vi "Window-Playback speed entry.vi"() -> (0 "error out":errorcluster, 2 "Frame rate set (fps)":dbl)   [LabVIEW 2013]
doc: "Use this template to create a dialog box with event handling."
uses:
  <vilib>/Utility/miscctls.llb/LVPointTypeDef.ctl
  Globals/gl_Time series viewer globals.vi
  Global Variables/General Globals.vi
panel:
  in  "Use custom FPS":bool
  out "Ind":dbl format="%#.1f FPS"
  in  "Playback speed (FPS)":dbl(slide)=10.0 caption="Playback speed" min=1.0 max=300.0 step=1.0 scale=1.0..300.0
  in  "Cancel":bool
  in  "OK":bool
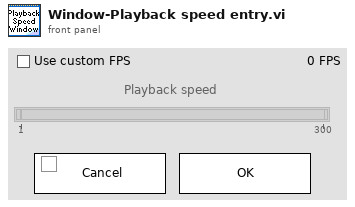
[diagram p1: front panel]
types:
  T1 = typedef "LVPointTypeDef.ctl" = cluster{"Horizontal":i16, "Vertical":i16}
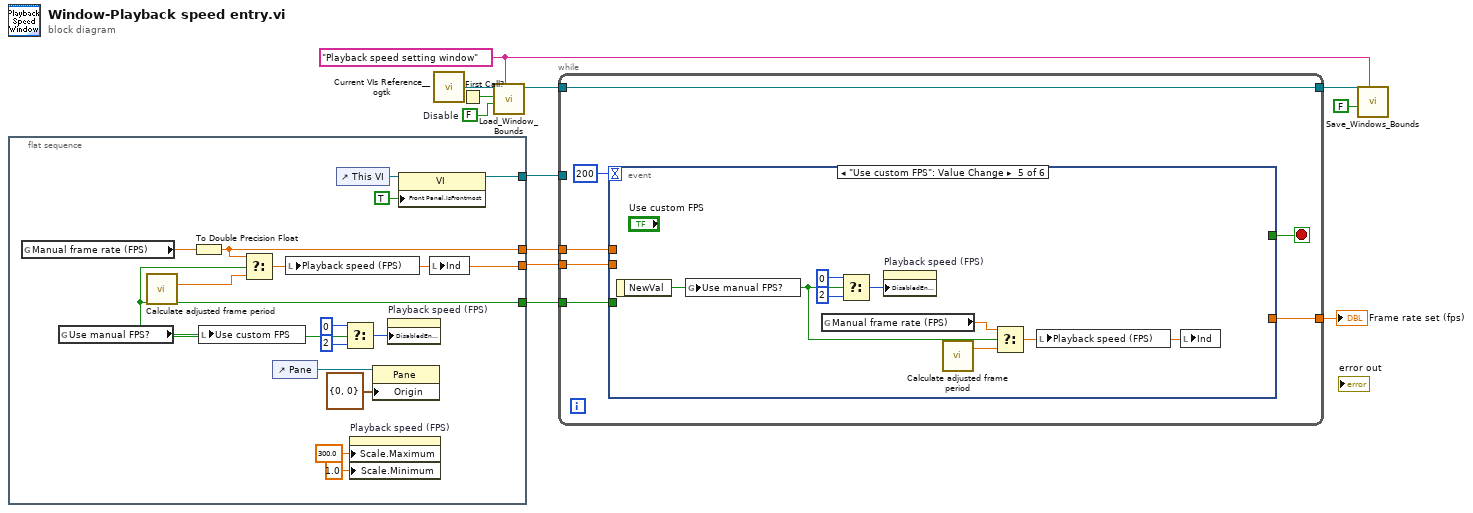
[diagram p0: block diagram]
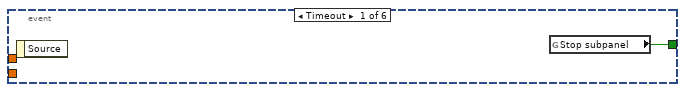
[diagram p2: hidden frame]
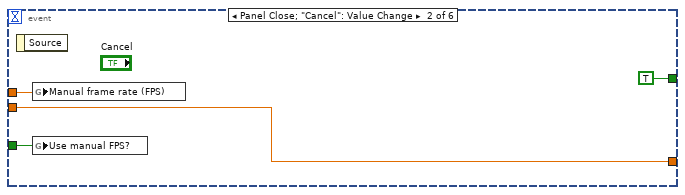
[diagram p3: hidden frame]
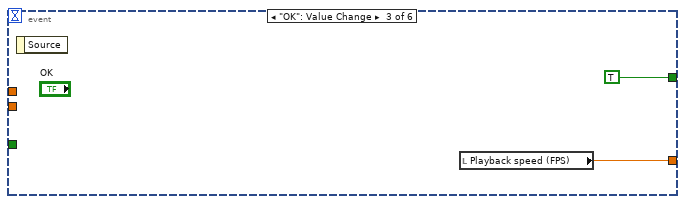
[diagram p4: hidden frame]
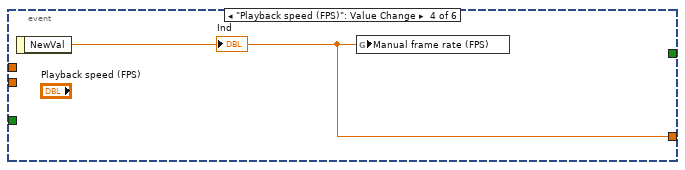
[diagram p5: hidden frame]
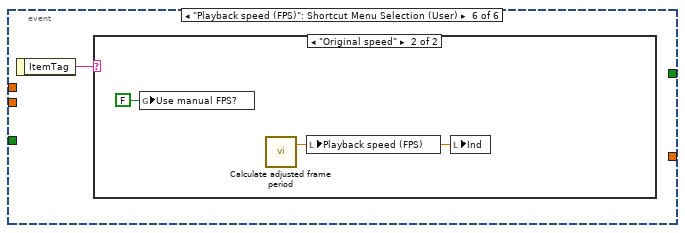
[diagram p6: hidden frame]
diagram:
  w8 = FALSE  # Disable
  w4 = "Playback speed setting window" ("Window Name (i.e. Key)")
  n1 = flat-sequence {
    tunnel: [w25] -> w12
    tunnel: [w17] -> w11
    tunnel: [w13] -> w2
    tunnel: [w15] -> w1
    frame #0 {
      n2 = global read "gl_Time series viewer globals.vi" "Manual frame rate (FPS)"() -> (w16:dbl)
      n3 = global read "gl_Time series viewer globals.vi" "Use manual FPS?"() -> (w15:bool)
      n4 = call "Calculate adjusted frame period.vi"() -> ("Original frame rate (fps)"=w14:dbl)  [unwired: 9 in, 2 out]
      n5 = To Double Precision Float(number=w16) -> (double precision float=w13:dbl)
      n6 = local write "Use custom FPS"(w15) -> ()
      n7 = Select(t=w13, s=w15, f=w14) -> (s? t:f=w17:dbl)
      n8 = control-ref of="Pane"() -> (w23:refnum<vi>)
      n9 = local write "Playback speed (FPS)"(w17) -> ()
      n10 = control-ref of="This VI"() -> (w26:refnum<vi>)
      n11 = Select(t=0, s=w15, f=2) -> (s? t:f=w18:i32)
      n12 = property on="Playback speed (FPS)" class="Slide (strict)"("Scale.Maximum"=300.0 ("Scale.Range:Maximum"), "Scale.Minimum"=1.0 ("Scale.Range:Minimum")) -> ()  [unwired: 2 in, 2 out]
      n13 = property class="Pane"(reference=w23, "Origin"=T1 {"Horizontal"=0, "Vertical"=0}) -> ()  [unwired: 1 in, 2 out]
      n14 = property on="Playback speed (FPS)" class="Slide (strict)"("DisabledEnum"=w18) -> ()  [unwired: 2 in, 2 out]
      n15 = property on="Property Node" class="VI"(reference=w26, "Front Panel.IsFrontmost"=TRUE ("Front Panel Window:Is Frontmost")) -> (reference out=w25:refnum<vi>)  [unwired: 1 in, 1 out]
      n16 = local write "Ind"(w17) -> ()
    }
  }
  n17 = call "Current VIs Reference__ogtk.vi"() -> ("Current VI's reference"=w10:refnum<vi>)  [unwired: 5 in]
  n18 = First Call?() -> (First Call?: T/F=w9:bool)
  n19 = call "Load_Window_Bounds.vi"("Window Name (i.e. Key)"=w4, "Disable"=w8, "First Call"=w9, "Window VI's Ref"=w10) -> ("reference out"=w6:refnum<vi>)  [unwired: 4 in, 3 out]
  n20 = while {
    tunnel: w12 -> [_]
    tunnel: w11 -> [w32]
    tunnel: w6 -> [w31]
    tunnel: [w31] -> w5
    tunnel: [w30] -> w3
    tunnel: w2 -> [w29]
    tunnel: w1 -> [w28]
    stop <- w34 stop-if-true
    n21 = event shown="[4] \"Use custom FPS\": Value Change" {
      selector: _ -> [_ _ _ _ _ _]
      dyn-events: _ -> [_ _ _ _ _ _]
      timeout: 200 -> [_ _ _ _ _ _]
      tunnel: [w35 TRUE ("Stop?") TRUE ("Stop?") _ _ _] -> w34
      tunnel: w32 -> [_ w38 _ _ _ _]
      tunnel: [_ w38 w40 w42 _ _] -> w30
      tunnel: w29 -> [_ w37 _ _ _ _]
      tunnel: w28 -> [_ w36 _ _ _ _]
      event Timeout {
        n22 = event-data() -> ()  [unwired: 1 in, 1 out]
        n23 = global read "General Globals.vi" "Stop subpanel"() -> (w35:bool)
      }
      event Panel Close; "Cancel": Value Change {
        n24 = event-data() -> ()  [unwired: 1 in, 1 out]
        n25 = global write "gl_Time series viewer globals.vi" "Manual frame rate (FPS)"(w37) -> ()
        n26 = global write "gl_Time series viewer globals.vi" "Use manual FPS?"(w36) -> ()
      }
      event "OK": Value Change {
        n27 = event-data() -> ()  [unwired: 1 in, 1 out]
        n28 = local read "Playback speed (FPS)"() -> (w40:dbl)
      }
      event "Playback speed (FPS)": Value Change {
        n29 = event-data() -> ("NewVal"=w42:dbl)  [unwired: 1 in]
        "Ind" <- w42
        n30 = global write "gl_Time series viewer globals.vi" "Manual frame rate (FPS)"(w42) -> ()
      }
      event "Use custom FPS": Value Change {
        n31 = event-data() -> ("NewVal"=w44:bool)  [unwired: 1 in]
        n32 = global write "gl_Time series viewer globals.vi" "Use manual FPS?"(w44) -> ()
        n33 = global read "gl_Time series viewer globals.vi" "Manual frame rate (FPS)"() -> (w45:dbl)
        n34 = Select(t=0, s=w44, f=2) -> (s? t:f=w49:i32)
        n35 = property on="Playback speed (FPS)" class="Slide (strict)"("DisabledEnum"=w49) -> ()  [unwired: 2 in, 2 out]
        n36 = call "Calculate adjusted frame period.vi"() -> ("Original frame rate (fps)"=w43:dbl)  [unwired: 9 in, 2 out]
        n37 = Select(t=w45, s=w44, f=w43) -> (s? t:f=w46:dbl)
        n38 = local write "Playback speed (FPS)"(w46) -> ()
        n39 = local write "Ind"(w46) -> ()
      }
      event "Playback speed (FPS)": Shortcut Menu Selection (User) {
        n40 = event-data() -> ("ItemTag"=w50:string)  [unwired: 1 in]
        n41 = case shown="\"Original speed\"" w50 {
          frame Default {
          }
          frame "Original speed" {
            n42 = global write "gl_Time series viewer globals.vi" "Use manual FPS?"(FALSE ("Use manual FPS?")) -> ()
            n43 = call "Calculate adjusted frame period.vi"() -> ("Original frame rate (fps)"=w51:dbl)  [unwired: 9 in, 2 out]
            n44 = local write "Playback speed (FPS)"(w51) -> ()
            n45 = local write "Ind"(w51) -> ()
          }
        }
      }
    }
  }
  "Frame rate set (fps)" <- w3
  n46 = call "Save_Windows_Bounds.vi"("Window Name (i.e. Key)"=w4, "Front Panel Window:Open"=FALSE, "Window VI's Ref"=w5) -> ()  [unwired: 8 in, 1 out]
